vi "licdf record read.vi"(6 "out_len":i32, 7 "out_cap":i32, 8 "error in (no error)":errorcluster, 9 "out":string, 10 "name":string, 11 "handle":i32) -> (0 "error out":errorcluster, 1 "out out":string, 3 "function return":i32, 4 "out_len out":i32)   [LabVIEW 2026, in "keynub_licdongle.lvlib"]
doc: "int32_t licdf_record_read(int32_t handle, const char *name, uint8_t *out, int32_t out_cap,\n int32_t *out_len);"
uses:
  keynub_licdongle.lvlib
  natives/win-x64/keynub_licdongle_flat.dll
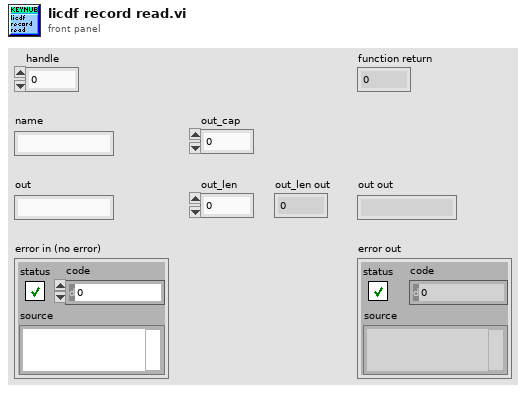
[diagram p1: front panel]
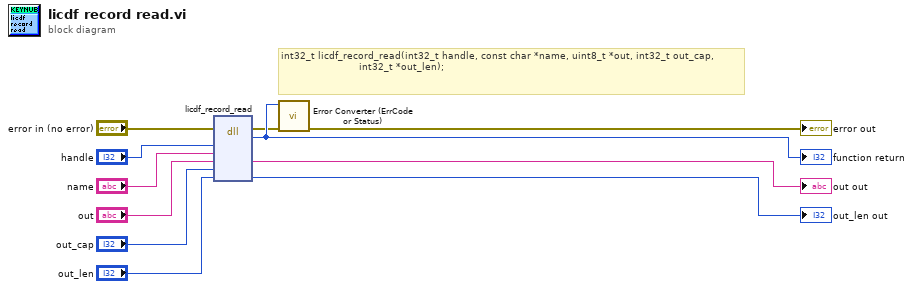
[diagram p0: block diagram]
diagram:
  # "int32_t licdf_record_read(int32_t handle, const char *name, uint8_t *out, int32_t out_cap,\n                          int32_t *out_len);"
  n1 = dll-call lib="C:/Austausch/KeyNub/LicenseDongle-PublicSDK/natives/win-x64/keynub_licdongle_flat.*" fn="licdf_record_read"(error in="error in (no error)", "handle"="handle", "name"="name", "out"="out", "out_cap"="out_cap", "out_len"="out_len") -> (error out=w2:errorcluster, w11:i32, "out"=→"out out":string, "out_len"=→"out_len out":i32)  [unwired: 5 in, 1 out]
  "function return" <- w11
  n2 = call "Error Converter (ErrCode or Status).vi"("error in (no error)"=w2, "error code"=w11) -> ("error out"=→"error out":errorcluster)  [unwired: 9 in]
